vi "Slave - Latency Simple.vi"() -> ()   [LabVIEW 2016]
uses:
  <vilib>/Utility/error.llb/DialogType.ctl
  <vilib>/Platform/TimedLoop/XDataNode/timing_clust.ctl
  <vilib>/Platform/TimedLoop/XDataNode/nitl_modes.ctl
  <vilib>/Platform/TimedLoop/XDataNode/wakeup.ctl
  <vilib>/pximc/Initialize Writer Session (DBL).vi
  <vilib>/pximc/Connect (DBL).vi
  <vilib>/pximc/Acquire Write Region (DBL).vi
  <vilib>/platform/TimedLoop/XDataNode/XDataNode.xnode
  <vilib>/pximc/nipximc.lvlib
  <vilib>/Platform/TimedLoop/XDataNode/XDNodeRunTimeDep.lvlib
panel:
  out "Latency":dbl format="%#.2p"
  out "Throughput S/s":dbl format="%#.2p"
  out "Time has Elapsed":bool
  in  "Stop Button":bool
  in  "#Writing Channels Slave 1":i32=2
  in  "Node 1 Writer Connection ID":u16=1
  in  "Node 1 Writer Interface":tag="PXIMC2" caption="interface"
  in  "Connection Timeout (s)":dbl=60.0 caption="timeout in seconds (-1)"
  # "Node 1"
  # "Node 2 => Node 1"
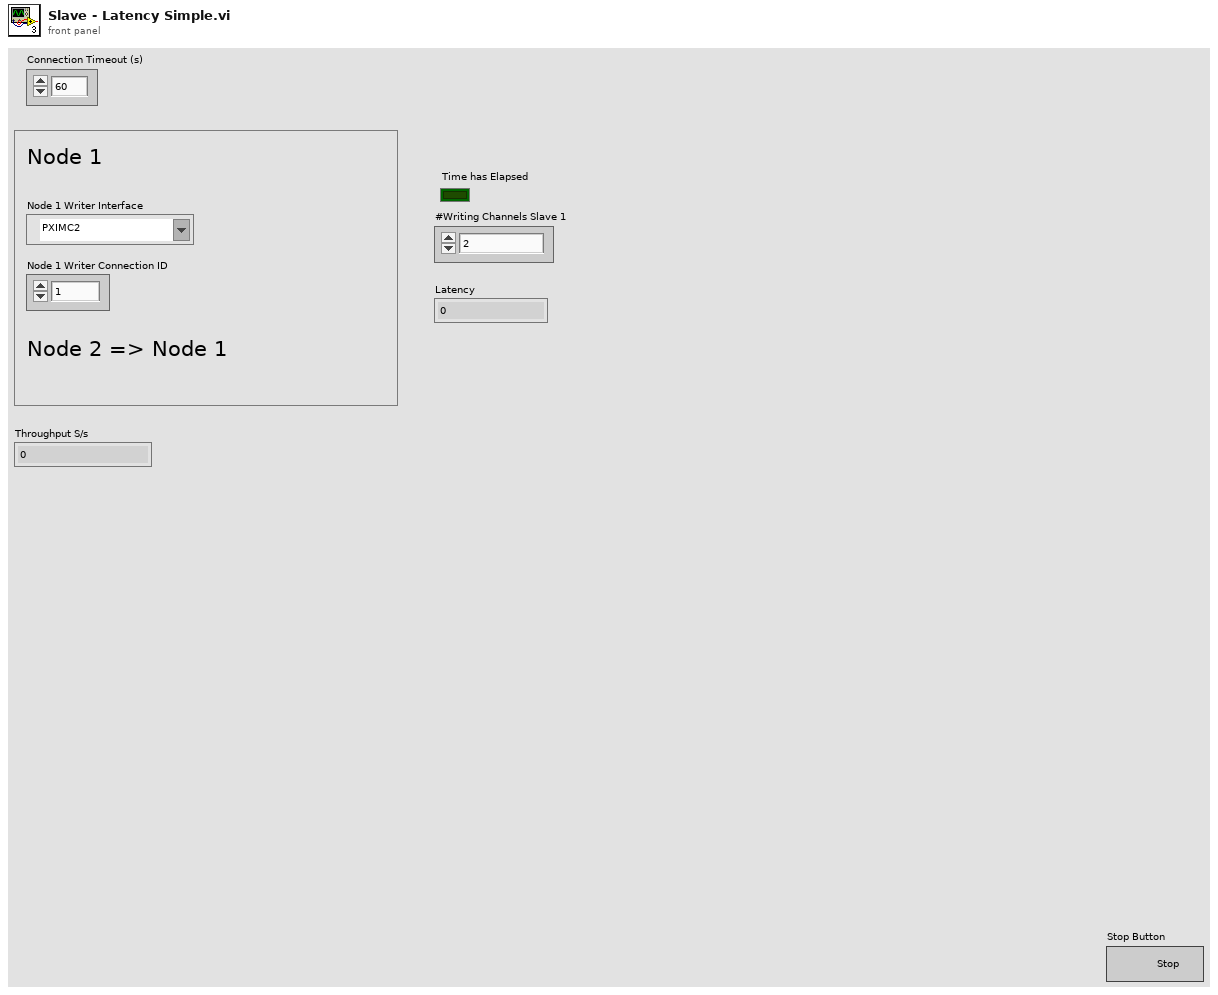
[diagram p1: front panel]
types:
  T1 = typedef "DialogType.ctl" = u16
  T2 = typedef "XDNodeRunTimeDep.lvlib/timing_clust.ctl" = cluster{"Expected End [f-1]":u64, "Actual End [f-1]":u64, "Finished Late? [f-1]":bool, "Expected End [i-1]":u64, "Actual End [i-1]":u64, "Finished Late? [i-1]":bool, "Expected Start [i]":u64, "Actual Start [i]":u64, "Expected Start [f]":u64, "Actual Start [f]":u64, "Source Name":string, "Structure Name":string, "Period":i64, "Deadline":i64, "Offset":i64, "Start":i64, "Priority":i32, "Timeout":i32, "Mode":T3, "Wakeup Reason":T4, "Error":errorcluster, "Source Type":string, "Secondary Source Type":string, "Global End Time":u64, "Global Start Time":u64, "Frame Duration":u64, "Iteration Duration":u64, "Assigned CPU":i32, "I/O Scan Engine Mode":u32}
  T3 = typedef "XDNodeRunTimeDep.lvlib/nitl_modes.ctl" = enum32{"No Change", "Process missed periods, maintain original phase", "Discard missed periods, maintain original phase", "Process missed periods, ignore original phase", "Discard missed periods, ignore original phase"}
  T4 = typedef "XDNodeRunTimeDep.lvlib/wakeup.ctl" = enum32{"Normal", "Aborted", "Asynchronous wakeup", "Timing source error", "Timed loop error", "Timeout"}
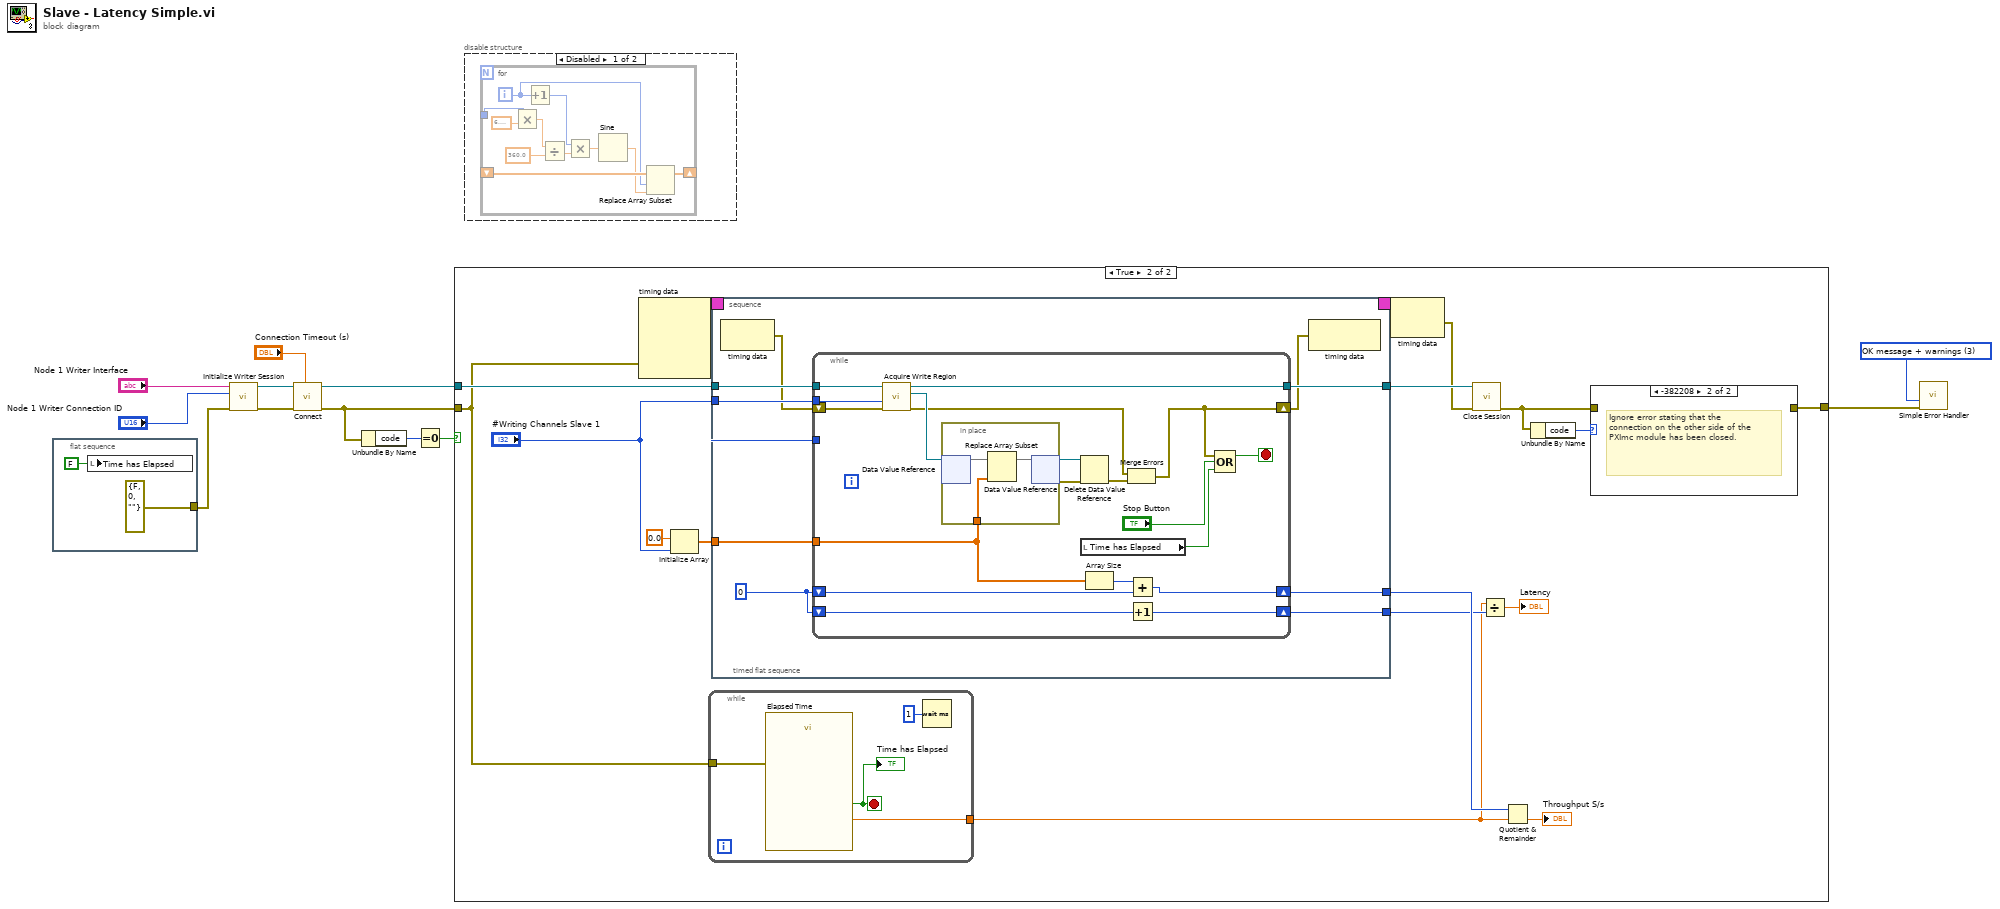
[diagram p0: block diagram]
diagram:
  w12 = T1 3 items=["no dialog", "OK message", "continue or stop message", "OK message + warnings", "continue/stop + warnings"] ("type of dialog (OK msg:1)")
  n1 = flat-sequence {
    tunnel: [errorcluster {"status"=FALSE, "code"=0, "source"=""} ("error constant")] -> w5
    frame #0 {
      n2 = local write "Time has Elapsed"(FALSE ("Stopped?")) -> ()
    }
  }
  n3 = call-poly <vilib>:"Initialize Writer Session.vi"("error in (no error)"=w5, "connection id (1)"="Node 1 Writer Connection ID", "interface"="Node 1 Writer Interface") -> ("error out"=w10:errorcluster, "session out"=w9:refnum<k21>)  [unwired: 7 in]
  n4 = call-poly <vilib>:"Connect.vi"("timeout in seconds (-1)"="Connection Timeout (s)", "error in (no error)"=w10, "session in"=w9) -> ("error out"=w1:errorcluster, "session out"=w6:refnum<k21>)  [unwired: 7 in]
  n5 = Unbundle By Name(w1) -> ("code"=w7:i32)
  n6 = Equal To 0?(x=w7) -> (x = 0?=w2:bool)
  n7 = case shown="True" w2 {
    tunnel: [w15 w32] -> w4
    tunnel: w6 -> [_ w30]
    tunnel: w1 -> [w15 w17]
    frame False {
      # "The connection was not successful for some reason."
    }
    frame True {
      n8 = node-c288(w17) -> (w19:T2)  [unwired: 3 in]
      n9 = Initialize Array(0.0 ("element"), "#Writing Channels Slave 1") -> (w24:dbl[])
      n10 = while {
        tunnel: w17 -> [w82]
        tunnel: [w81] -> w21
        stop <- w83 stop-if-true
        n11 = call "Elapsed Time"("error in (no error)"=w82) -> ("Elapsed Time (s)"=w81:dbl, "Time has Elapsed"=w83:bool)  [unwired: 11 in, 6 out]
        "Time has Elapsed" <- w83
        n12 = Wait (ms)(milliseconds to wait=u32 1) -> ()  [unwired: 1 out]
      }
      n13 = timed-sequence {
        timing: w19 -> [_]
        timing-out: [_] -> w18
        tunnel: w30 -> [w38]
        tunnel: [w37] -> w29
        tunnel: [w36] -> w27
        tunnel: w24 -> [w35]
        tunnel: "#Writing Channels Slave 1" -> [w34]
        tunnel: [w33] -> w22
        n14 = timed-flat-sequence {
          tunnel: w38 -> [w47]
          tunnel: [w46] -> w37
          tunnel: [w45] -> w36
          tunnel: w35 -> [w44]
          tunnel: w34 -> [w43]
          tunnel: [w41] -> w33
          w42 = u32 0 ("element")
          n15 = node-c288() -> (w40:errorcluster)  [unwired: 1 in]
          n16 = while {
            tunnel: w47 -> [w61]
            tunnel: [w60] -> w46
            shift-right: [w58] -> w39
            shift-left: w40 -> [w59]
            shift-right: [w54] -> w45
            shift-left: w42 -> [w55]
            tunnel: w44 -> [w50]
            tunnel: w43 -> [w51]
            tunnel: w43 -> [_]
            shift-right: [w48] -> w41
            shift-left: w42 -> [w49]
            stop <- w57 stop-if-true
            n17 = call-poly <vilib>:"Acquire Write Region.vi"("error in (no error)"=w59, "number of elements"=w51, "session in"=w61) -> ("error out"=w62:errorcluster, "write region reference"=w63:refnum<data-value>, "session out"=w60:refnum<k21>)  [unwired: 5 in, 1 out]
            n18 = in-place {
              in-place-border: w50 -> [w67]
              n19 = in-place-dvr #1(w63) -> (w69:dbl[])  [unwired: 1 out]
              n20 = Replace Array Subset(array=w69, new element=w67) -> (w68:dbl[])  [unwired: 1 in]
              n21 = in-place-dvr #1(w68) -> (w64:refnum<data-value>, w66:errorcluster)
            }
            n22 = Delete Data Value Reference(data value reference=w64, error in=w66) -> (error out=w65:errorcluster)  [unwired: 1 out]
            n23 = local read "Time has Elapsed"() -> (w53:bool)
            n24 = Array Size(array=w50) -> (size(s)=w52:i32)
            n25 = Merge Errors(w62, w65) -> (w58:errorcluster)
            n26 = Add(x=w52, y=w55) -> (x+y=w54:u32)
            n27 = Increment(x=w49) -> (x+1=w48:u32)
            n28 = Compound Arithmetic op=OR(w58, "Stop Button", w53) -> (w57:bool)
          }
          n29 = node-c288(w39) -> ()  [unwired: 1 out]
        }
      }
      n30 = node-c288(w18) -> (w16:errorcluster)
      n31 = call <vilib>:"Close Session.vi"("error in (no error)"=w16, "session in"=w29) -> ("error out"=w28:errorcluster)  [unwired: 9 in]
      n32 = Divide(x=w21, y=w22) -> (x/y=→"Latency":dbl)
      n33 = Quotient & Remainder(x=w27, y=w21) -> (floor(x/y)=→"Throughput S/s":dbl)  [unwired: 1 out]
      n34 = Unbundle By Name(w28) -> ("code"=w31:i32)
      n35 = case shown="-382208" w31 {
        tunnel: w28 -> [w84 _]
        tunnel: [w84 _] -> w32
        frame 0, Default {
        }
        frame -382208 {
          # "Ignore error stating that the connection on the other side of the PXImc module has been closed."
        }
      }
    }
  }
  n36 = disable-structure shown="Disabled" {
    frame Disabled {
      n37 = for {
        tunnel: _ -> [w89]
        shift-right: [w87] -> _
        shift-left: _ -> [w88]
        i -> [w85]
        n38 = Multiply(x=w89, y=6.283185307179586) -> (x*y=w92:dbl)
        n39 = Increment(x=w85) -> (x+1=w90:i32)
        n40 = Divide(x=w92, y=360.0) -> (x/y=w94:dbl)
        n41 = Multiply(x=w90, y=w94) -> (x*y=w95:dbl)
        n42 = Sine(x=w95) -> (sin(x)=w86:dbl)
        n43 = Replace Array Subset(array=w88, new element=w86, index=w85) -> (w87:dbl[])
      }
    }
    frame Enabled {
    }
  }
  n44 = call <vilib>:"Simple Error Handler.vi"("type of dialog (OK msg:1)"=w12, "error in (no error)"=w4) -> ()  [unwired: 3 in, 5 out]
